vi "addzero.vi"(11 "?":string="21") -> (1 "String 2":string)   [LabVIEW 2022 SP3]
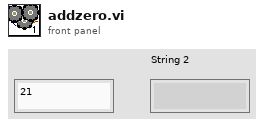
[diagram p1: front panel]
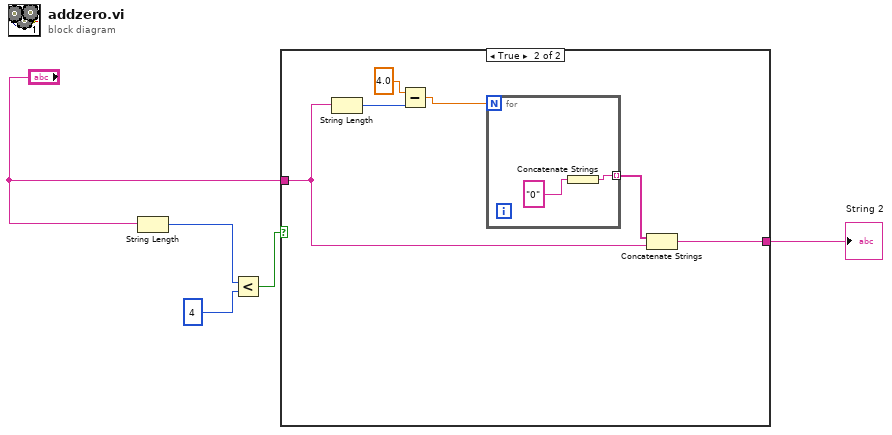
[diagram p0: block diagram]
diagram:
  n1 = String Length(string="?") -> (length=w4:i32)
  n2 = Less?(x=w4, y=4) -> (x < y?=w3:bool)
  n3 = case shown="True" w3 {
    tunnel: "?" -> [w6 w8]
    tunnel: [w6 w7] -> w2
    frame False {
    }
    frame True {
      n4 = String Length(string=w8) -> (length=w12:i32)
      n5 = Subtract(x=4.0, y=w12) -> (x-y=w10:dbl)
      n6 = for {
        N: w10 -> [_]
        tunnel: [w13] -> w9 mode=indexing
        n7 = Concatenate Strings("0") -> (w13:string)
      }
      n8 = Concatenate Strings(w9, w8) -> (w7:string)
    }
  }
  "String 2" <- w2
